vi "Test Lockin Digitizer with Counter.vi"(8 "error in":errorcluster) -> ()   [LabVIEW 2021]
uses:
  <vilib>/DAQmx/write.llb/DAQmx Write (Analog 1D DBL 1Chan NSamp).vi
  <vilib>/DAQmx/read.llb/DAQmx Read (Analog 1D DBL 1Chan NSamp).vi
  <vilib>/DAQmx/create/channels.llb/DAQmx Create Channel (AO-Voltage-Basic).vi
  <vilib>/DAQmx/create/channels.llb/DAQmx Create Channel (CO-Pulse Generation-Frequency).vi
  <vilib>/DAQmx/configure/timing.llb/DAQmx Timing (Implicit).vi
  <vilib>/DAQmx/create/channels.llb/DAQmx Create Channel (AI-Voltage-Basic).vi
  <vilib>/DAQmx/configure/timing.llb/DAQmx Timing (Sample Clock).vi
  <vilib>/DAQmx/miscellaneous.llb/DAQmx Fill In Error Info.vi
  <vilib>/DAQmx/configure/trigger.llb/DAQmx Reference Trigger (Digital Edge).vi
  <resource>/objmgr/daqmx.rc
  <vilib>/Analysis/NI_AALBase.lvlib
panel:
  out "x/y":dbl
  out "CO.Count":u32
  out "CO.CtrTimebaseRate":dbl format="%#_6p"
  in  "AI samples per channel":i32=1000
  out "Waveform Graph":dbl[](graph)
  in  "Buffer":i32=128
  in  "AI chan":tag
  out "Actual sample rate":dbl format="%#_6p"
  in  "AO chan":tag
  in  "pretrigger samples per channel":u32=500
  out "Done":bool
  in  "Stop Button":bool
  in  "Trigger source":tag
  in  "Desired sample rate":dbl=96.0 format="%#_6pHz"
  in  "counter":tag
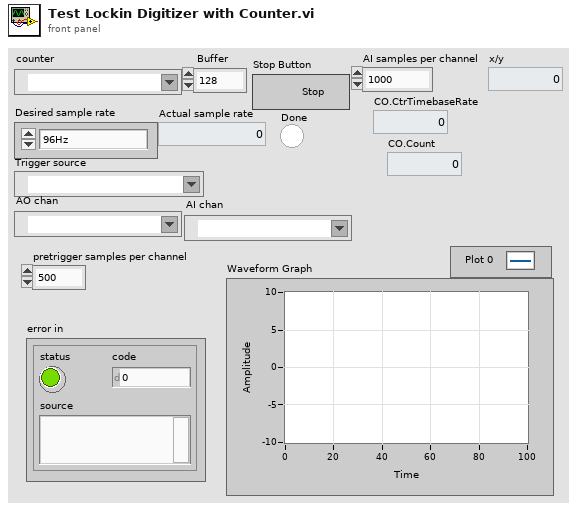
[diagram p1: front panel]
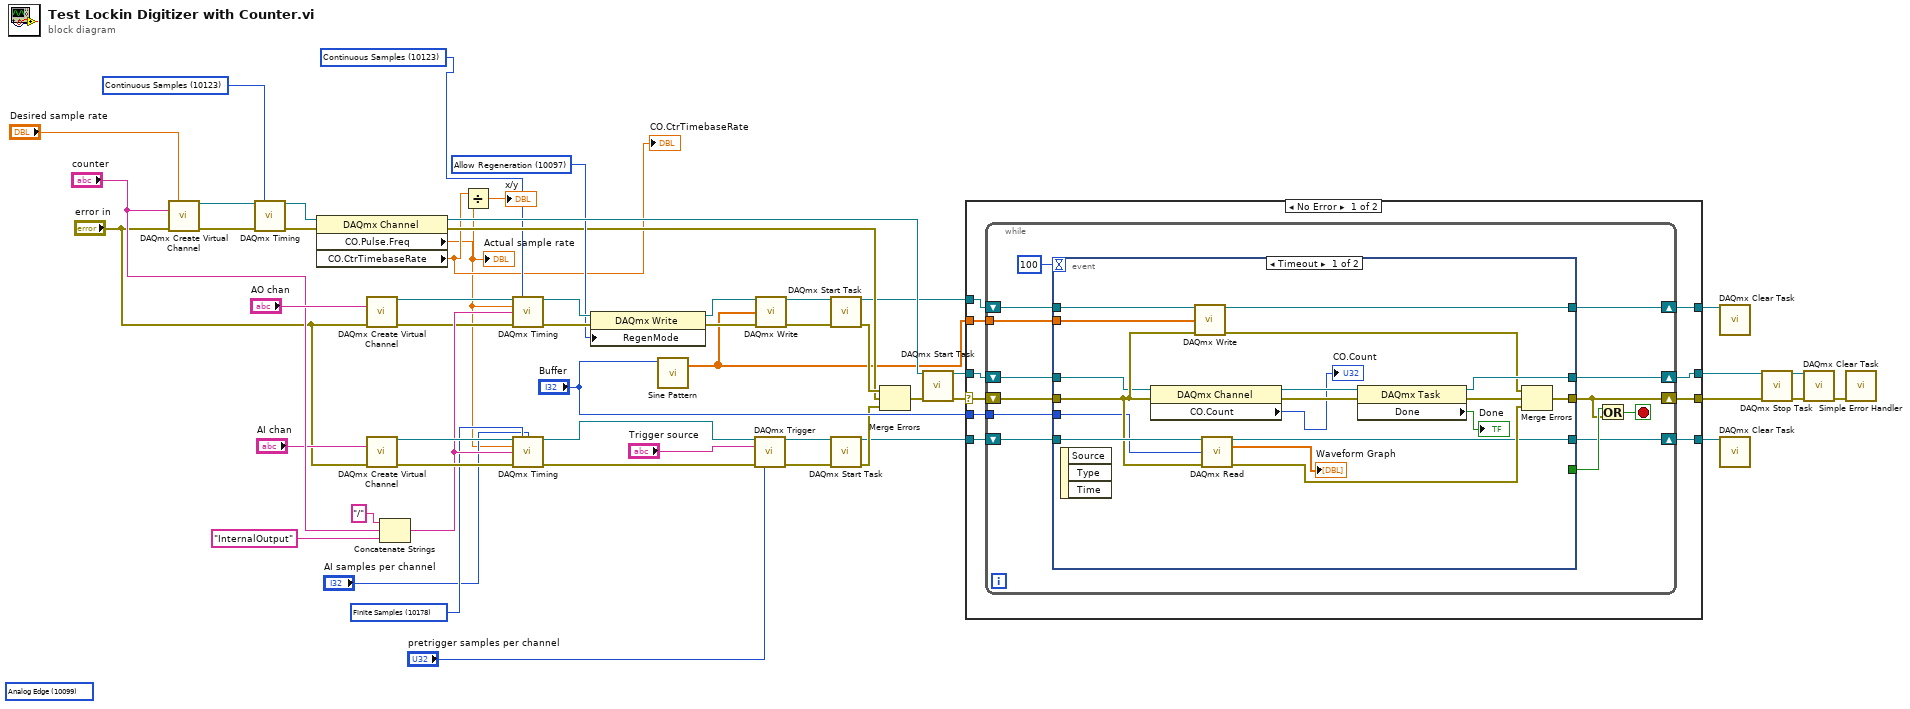
[diagram p0: block diagram]
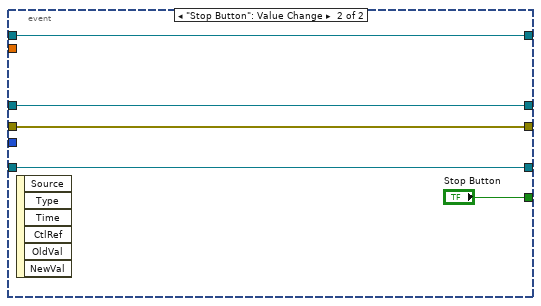
[diagram p2: hidden frame]
diagram:
  w12 = 10123 items=["Finite Samples"=10178, "Continuous Samples"=10123, "Hardware Timed Single Point"=12522] ("sample mode")
  w13 = 10178 items=["Finite Samples"=10178, "Continuous Samples"=10123, "Hardware Timed Single Point"=12522] ("sample mode")
  w34 = 10097 items=["Allow Regeneration"=10097, "Do Not Allow Regeneration"=10158] ("RegenMode")
  w52 = 10123 items=["Finite Samples"=10178, "Continuous Samples"=10123, "Hardware Timed Single Point"=12522] ("sample mode")
  (unwired) 10099 items=["Analog Edge"=10099, "Analog Multi Edge"=16108, "Digital Edge"=10150, "Digital Pattern"=10398, "Analog Window"=10103, "Time"=15996, "None"=10230] ("Start.TrigType")
  n1 = call-poly <vilib>:"DAQmx Create Virtual Channel.vi"("frequency"="Desired sample rate", "counter"="counter", "error in"="error in") -> ("task out"=w53:refnum<k21>, "error out"=w54:errorcluster)  [unwired: 11 in]
  n2 = call-poly <vilib>:"DAQmx Timing.vi"("task/channels in"=w53, "sample mode"=w52, "error in"=w54) -> ("task out"=w39:refnum<k21>, "error out"=w37:errorcluster)  [unwired: 11 in]
  n3 = property class="DAQmx Channel"(reference=w39, error in=w37) -> (reference out=w38:refnum<k21>, error out=w21:errorcluster, "CO.Pulse.Freq"=w2:dbl, "CO.CtrTimebaseRate"=w3:dbl)
  "Actual sample rate" <- w2
  "CO.CtrTimebaseRate" <- w3
  n4 = call-poly <vilib>:"DAQmx Create Virtual Channel.vi"("physical channels"="AO chan", "error in"="error in") -> ("task out"=w43:refnum<k21>, "error out"=w23:errorcluster)  [unwired: 12 in]
  n5 = call-poly <vilib>:"DAQmx Create Virtual Channel.vi"("physical channels"="AI chan", "error in"="error in") -> ("task out"=w30:refnum<k21>, "error out"=w29:errorcluster)  [unwired: 12 in]
  n6 = Concatenate Strings("/", "counter", "InternalOutput" ("string")) -> (w28:string)
  n7 = Divide(x=w3, y=w2) -> (x/y=→"x/y":dbl)
  n8 = call-poly <vilib>:"DAQmx Timing.vi"("task/channels in"=w43, "sample mode"=w12, "rate"=w2, "source"=w28, "error in"=w23) -> ("task out"=w35:refnum<k21>, "error out"=w36:errorcluster)  [unwired: 9 in]
  n9 = call-poly <vilib>:"DAQmx Timing.vi"("task/channels in"=w30, "sample mode"=w13, "samples per channel"="AI samples per channel", "rate"=w2, "source"=w28, "error in"=w29) -> ("task out"=w26:refnum<k21>, "error out"=w27:errorcluster)  [unwired: 8 in]
  n10 = property class="DAQmx Write"(reference=w35, error in=w36, "RegenMode"=w34) -> (reference out=w17:refnum<k21>, error out=w16:errorcluster)
  n11 = call <vilib>:"Sine Pattern.vi"("samples"="Buffer") -> ("Sinusoidal Pattern"=w14:dbl[])  [unwired: 3 in, 1 out]
  n12 = call-poly <vilib>:"DAQmx Trigger.vi"("task/channels in"=w26, "source"="Trigger source", "error in"=w27, "pretrigger samples per channel"="pretrigger samples per channel") -> ("task out"=w7:refnum<k21>, "error out"=w6:errorcluster)  [unwired: 10 in]
  n13 = call-poly <vilib>:"DAQmx Write.vi"("task/channels in"=w17, "data"=w14, "error in"=w16) -> ("task out"=w18:refnum<k21>, "error out"=w19:errorcluster)  [unwired: 10 in, 1 out]
  n14 = call <vilib>:"DAQmx Start Task.vi"("task/channels in"=w18, "error in"=w19) -> ("task out"=w20:refnum<k21>, "error out"=w33:errorcluster)  [unwired: 12 in]
  n15 = call <vilib>:"DAQmx Start Task.vi"("task/channels in"=w7, "error in"=w6) -> ("task out"=w4:refnum<k21>, "error out"=w5:errorcluster)  [unwired: 12 in]
  n16 = Merge Errors(w33, w21, w5) -> (w22:errorcluster)
  n17 = call <vilib>:"DAQmx Start Task.vi"("task/channels in"=w38, "error in"=w22) -> ("task out"=w50:refnum<k21>, "error out"=w10:errorcluster)  [unwired: 12 in]
  n18 = case shown="No Error" w10 {
    selector: w10 -> [w57 w104]
    tunnel: w50 -> [w64 w103]
    tunnel: [w63 w103] -> w49
    tunnel: [w62 w104] -> w48
    tunnel: w20 -> [w61 w102]
    tunnel: w4 -> [w60 w101]
    tunnel: "Buffer" -> [w59 _]
    tunnel: w14 -> [w58 _]
    tunnel: [w56 w102] -> w9
    tunnel: [w55 w101] -> w8
    frame No Error {
      n19 = while {
        shift-right: [w74] -> w63
        shift-left: w64 -> [w75]
        shift-right: [w71] -> w62
        shift-left: w57 -> [w73]
        shift-right: [w69] -> w56
        shift-left: w61 -> [w70]
        shift-right: [w67] -> w55
        shift-left: w60 -> [w68]
        tunnel: w59 -> [w66]
        tunnel: w58 -> [w65]
        stop <- w72 stop-if-true
        n20 = event shown="[0] Timeout" {
          selector: _ -> [_ _]
          dyn-events: _ -> [_ _]
          timeout: 100 -> [_ _]
          tunnel: [_ "Stop Button"] -> w77
          tunnel: w75 -> [w79 w98]
          tunnel: [w95 w98] -> w74
          tunnel: w73 -> [w85 w97]
          tunnel: [w89 w97] -> w71
          tunnel: w70 -> [w90 w99]
          tunnel: [w87 w99] -> w69
          tunnel: w68 -> [w86 w96]
          tunnel: [w83 w96] -> w67
          tunnel: w66 -> [w82 _]
          tunnel: w65 -> [w80 _]
          event Timeout {
            n21 = event-data() -> ()  [unwired: 1 in, 3 out]
            n22 = property class="DAQmx Channel"(reference=w79, error in=w85) -> (reference out=w92:refnum<k21>, error out=w91:errorcluster, "CO.Count"=→"CO.Count":u32)
            n23 = call-poly <vilib>:"DAQmx Write.vi"("task/channels in"=w90, "data"=w80, "error in"=w85) -> ("task out"=w87:refnum<k21>, "error out"=w88:errorcluster)  [unwired: 10 in, 1 out]
            n24 = call-poly <vilib>:"DAQmx Read.vi"("task/channels in"=w86, "number of samples per channel"=w82, "error in"=w85) -> ("task out"=w83:refnum<k21>, "data"=→"Waveform Graph":dbl[], "error out"=w84:errorcluster)  [unwired: 10 in]
            n25 = property class="DAQmx Task"(reference=w92, error in=w91) -> (reference out=w95:refnum<k21>, error out=w94:errorcluster, "Done"=→"Done":bool)
            n26 = Merge Errors(w88, w94, w84) -> (w89:errorcluster)
          }
          event "Stop Button": Value Change {
            n27 = event-data() -> ()  [unwired: 1 in, 6 out]
          }
        }
        n28 = Or(x=w77, y=w71) -> (x .or. y?=w72:bool)
      }
    }
    frame Error {
    }
  }
  n29 = call <vilib>:"DAQmx Clear Task.vi"("task in"=w9) -> ()  [unwired: 14 in, 1 out]
  n30 = call <vilib>:"DAQmx Clear Task.vi"("task in"=w8) -> ()  [unwired: 14 in, 1 out]
  n31 = call <vilib>:"DAQmx Stop Task.vi"("task/channels in"=w49, "error in"=w48) -> ("task out"=w47:refnum<k21>, "error out"=w46:errorcluster)  [unwired: 12 in]
  n32 = call <vilib>:"DAQmx Clear Task.vi"("task in"=w47, "error in"=w46) -> ("error out"=w45:errorcluster)  [unwired: 13 in]
  n33 = call <vilib>:"Simple Error Handler.vi"("error in (no error)"=w45) -> ()  [unwired: 4 in, 5 out]
